vi "Sort Triangles.vi"(11 "Triangles":T1[](array[typedef]) {"Vertex 3"."UV"."v" min=0 max=1 step=0.1; "Vertex 3"."UV"."u" min=0 max=1 step=0.1; "Vertex 2"."UV"."v" min=0 max=1 step=0.1; "Vertex 2"."UV"."u" min=0 max=1 step=0.1; "Vertex 1"."UV"."v" min=0 max=1 step=0.1; "Vertex 1"."UV"."u" min=0 max=1 step=0.1}) -> (3 "Triangles Sorted":T1[](array[typedef]) {"Vertex 3"."UV"."v" min=0 max=1 step=0.1; "Vertex 3"."UV"."u" min=0 max=1 step=0.1; "Vertex 2"."UV"."v" min=0 max=1 step=0.1; "Vertex 2"."UV"."u" min=0 max=1 step=0.1; "Vertex 1"."UV"."v" min=0 max=1 step=0.1; "Vertex 1"."UV"."u" min=0 max=1 step=0.1})   [LabVIEW 2020, in "3D.lvlib"]
uses:
  3D.lvlib
  <userlib>/_OpenG.lib/array/array.llb/openg_array.lvlib
  <userlib>/_OpenG.lib/array/array.llb/Sort 1D Array (SGL)__ogtk.vi
  Vector 3D.ctl
  Raster/UV.ctl
  Raster/Raster.lvlib
  Vertex.ctl
  Triangle.ctl
  Raster/Rectangle Dimensions.ctl
  Raster/Texture.ctl
  Material.ctl
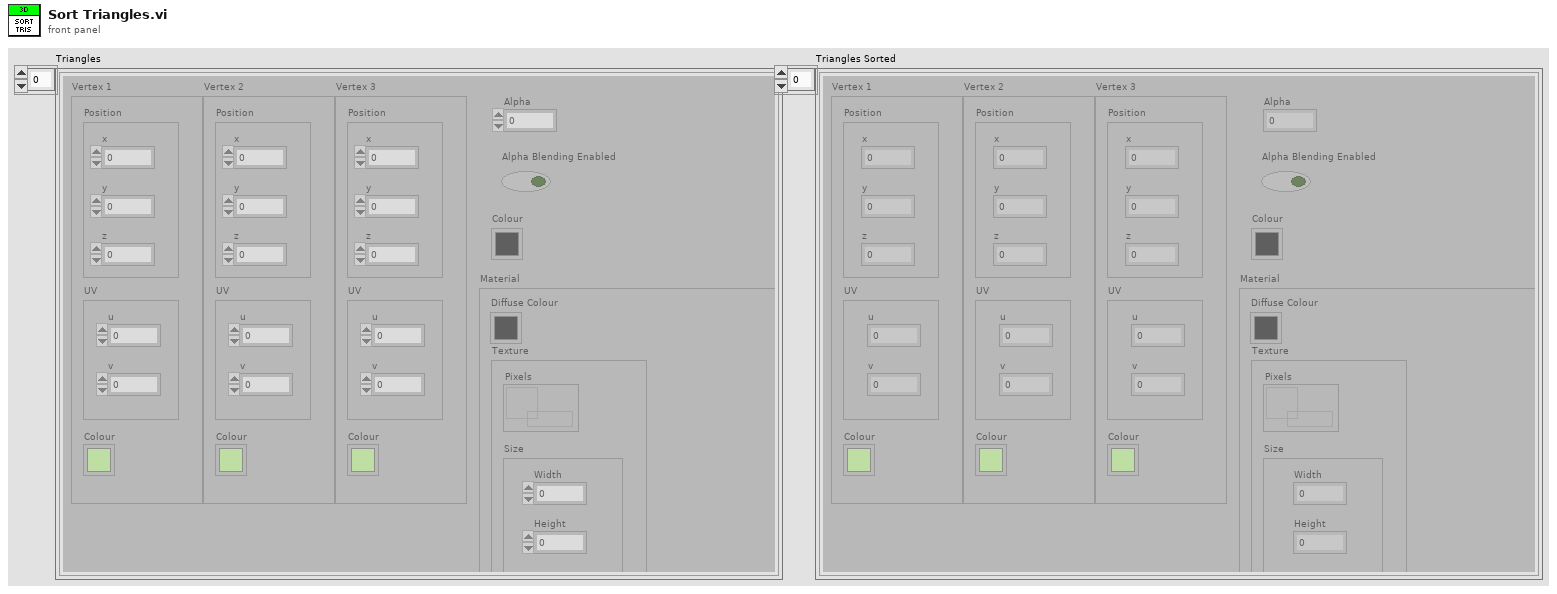
[diagram p1: front panel]
types:
  T1 = typedef "3D.lvlib/Triangle.ctl" = cluster{"Vertex 1":T2, "Vertex 2":T2, "Vertex 3":T2, "Alpha":dbl, "Alpha Blending Enabled":bool, "Colour":u32, "Material":T5}
  T2 = typedef "3D.lvlib/Vertex.ctl" = cluster{"Position":T3, "UV":T4, "Colour":u32}
  T3 = typedef "3D.lvlib/Vector 3D.ctl" = cluster{"x":sgl, "y":sgl, "z":sgl}
  T4 = typedef "Raster.lvlib/UV.ctl" = cluster{"u":sgl, "v":sgl}
  T5 = typedef "3D.lvlib/Material.ctl" = cluster{"Diffuse Colour":u32, "Texture":T6}
  T6 = typedef "Raster.lvlib/Texture.ctl" = cluster{"Pixels":refnum<data-value>, "Size":T7}
  T7 = typedef "Raster.lvlib/Rectangle Dimensions.ctl" = cluster{"Width":u32, "Height":u32}
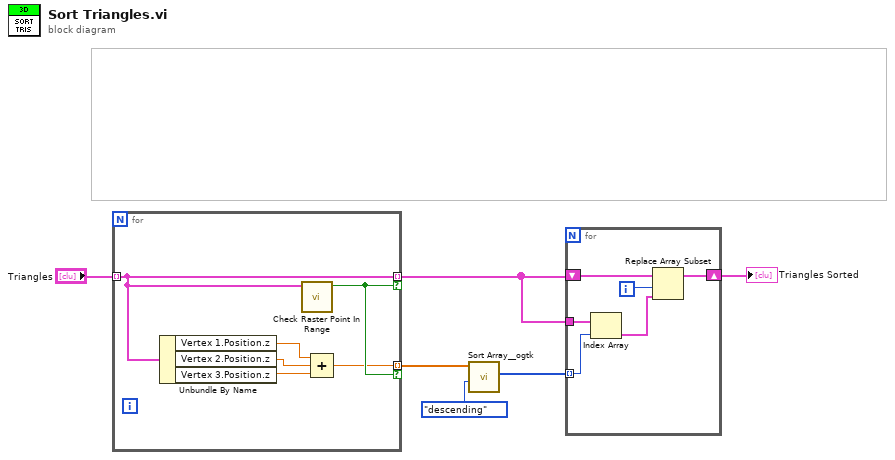
[diagram p0: block diagram]
diagram:
  n1 = for {
    tunnel: "Triangles" -> [w7] mode=indexing
    tunnel: [w7] -> w1 mode=indexing if=w12
    tunnel: [w11] -> w5 mode=indexing if=w12
    n2 = Unbundle By Name(w7) -> ("Vertex 1.Position.z"=w10:sgl, "Vertex 2.Position.z"=w9:sgl, "Vertex 3.Position.z"=w8:sgl)
    n3 = call "Check Raster Point In Range.vi"("Projected Triangle"=w7) -> ("Keep"=w12:bool)  [unwired: 10 in]
    n4 = Compound Arithmetic op=ADD(w10, w9, w8) -> (w11:sgl)
  }
  n5 = call-poly <userlib>:"Sort Array__ogtk.vi"("Order"=enum16{"ascending", "descending"}."descending", "Array in"=w5) -> ("Sorted Pointers"=w4:i32[])  [unwired: 8 in, 1 out]
  n6 = for {
    tunnel: w4 -> [w14] mode=indexing
    shift-right: [w16] -> w2
    shift-left: w1 -> [w17]
    tunnel: w1 -> [w15]
    i -> [w18]
    n7 = Index Array(array=w15, index=w14) -> (element=w13:T1)
    n8 = Replace Array Subset(array=w17, new element=w13, index=w18) -> (w16:T1[])
  }
  "Triangles Sorted" <- w2
